vi "Automatic CE-CERT Inverter MODBUS TCP-IP Curtailment.vi"() -> ()   [LabVIEW 2018]
uses:
  09a05df4-458d-4fd2-9c33-f3dfa60df926.vi
  86d118a4-68e0-4187-aa54-a9d0a6fa2209.vi
  7d9401a8-d984-499b-98ba-350348555d74.vi
  1c5b115a-7472-46f7-9b4a-cb66c2e2ccef.vi
  14952779-31b7-4685-9780-957b5950c005.vi
  aad8307b-7fea-461e-ba7f-5a63a8c7236a.vi
  df043d8b-bec8-4485-823e-7a72ed92ff53.vi
  6303200c-3b40-4aff-b068-1284407d55db.vi
  <vilib>/Plasmionique/MB Master/MB_Master_TCP/MB_Master_TCP.lvclass
  C:/Program Files (x86)/National Instruments/LabVIEW 2018/vi.lib/Plasmionique/MB Master/MB_Master/MB_Master.lvclass
  <vilib>/Plasmionique/MB Master/MB Master.lvlib
panel:
  in  "Stop Button":bool
  in  "Send Curtailment":bool
  out "Eighth Step Time (ms)":u32
  out "Seventh Step Time (ms)":u32
  out "Sixth Step Time (ms)":u32
  out "Fifth Step Time (ms)":u32
  out "Fourth Step Time (ms)":u32
  out "Third Step Time (ms)":u32
  out "Second Step Time (ms)":u32
  out "First Step Time (ms)":u32
  out "Program Runtime (ms)":u32
  in  "Curtailment Value (28-100%)":u16
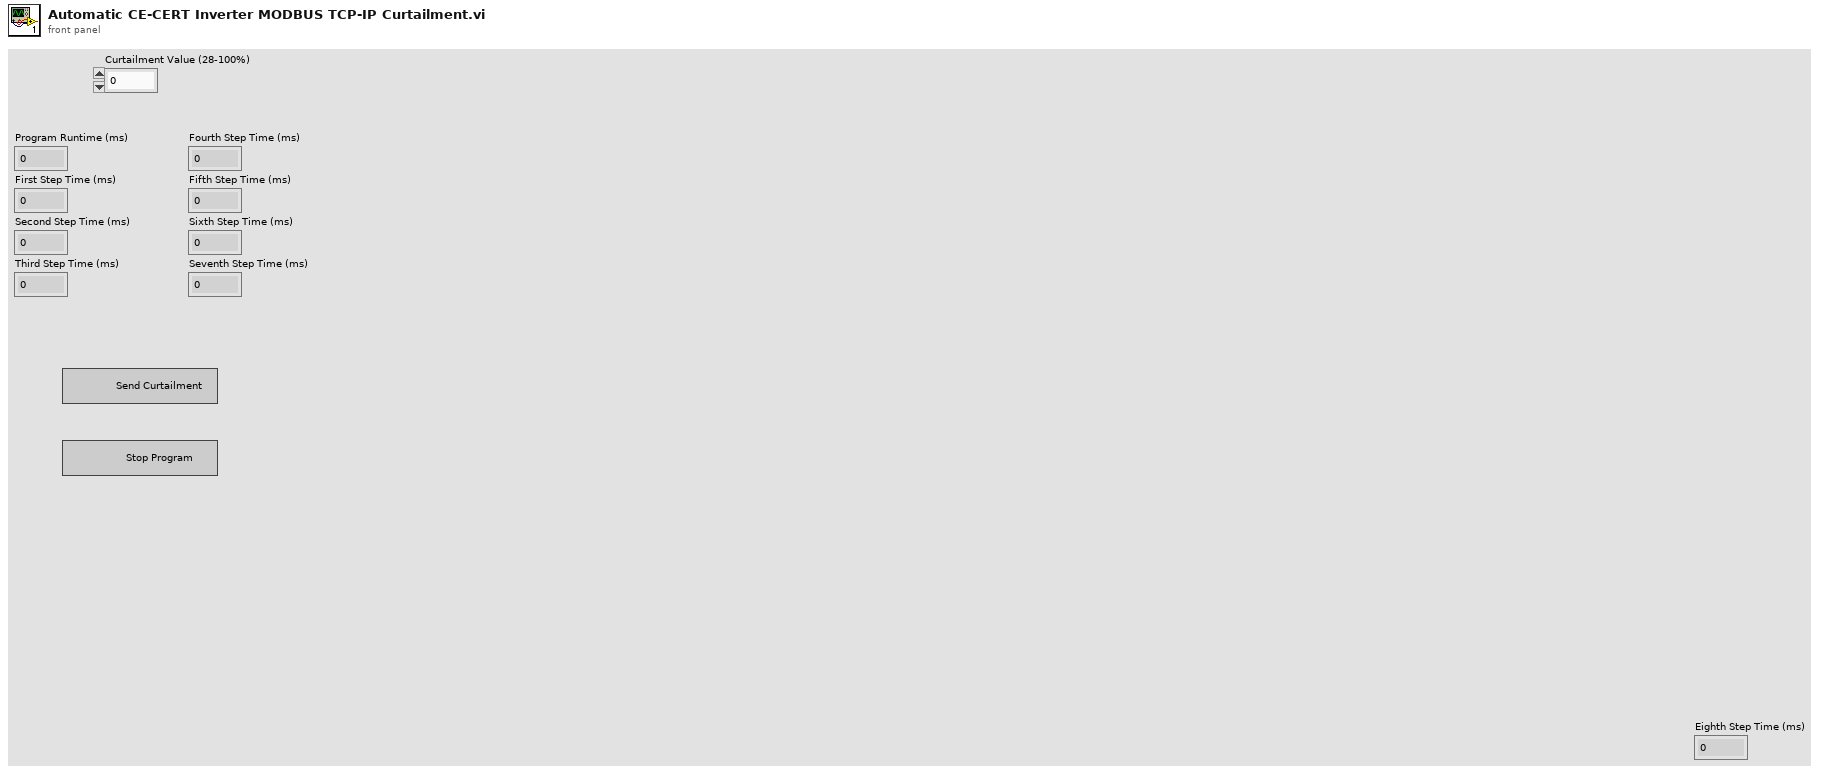
[diagram p1: front panel]
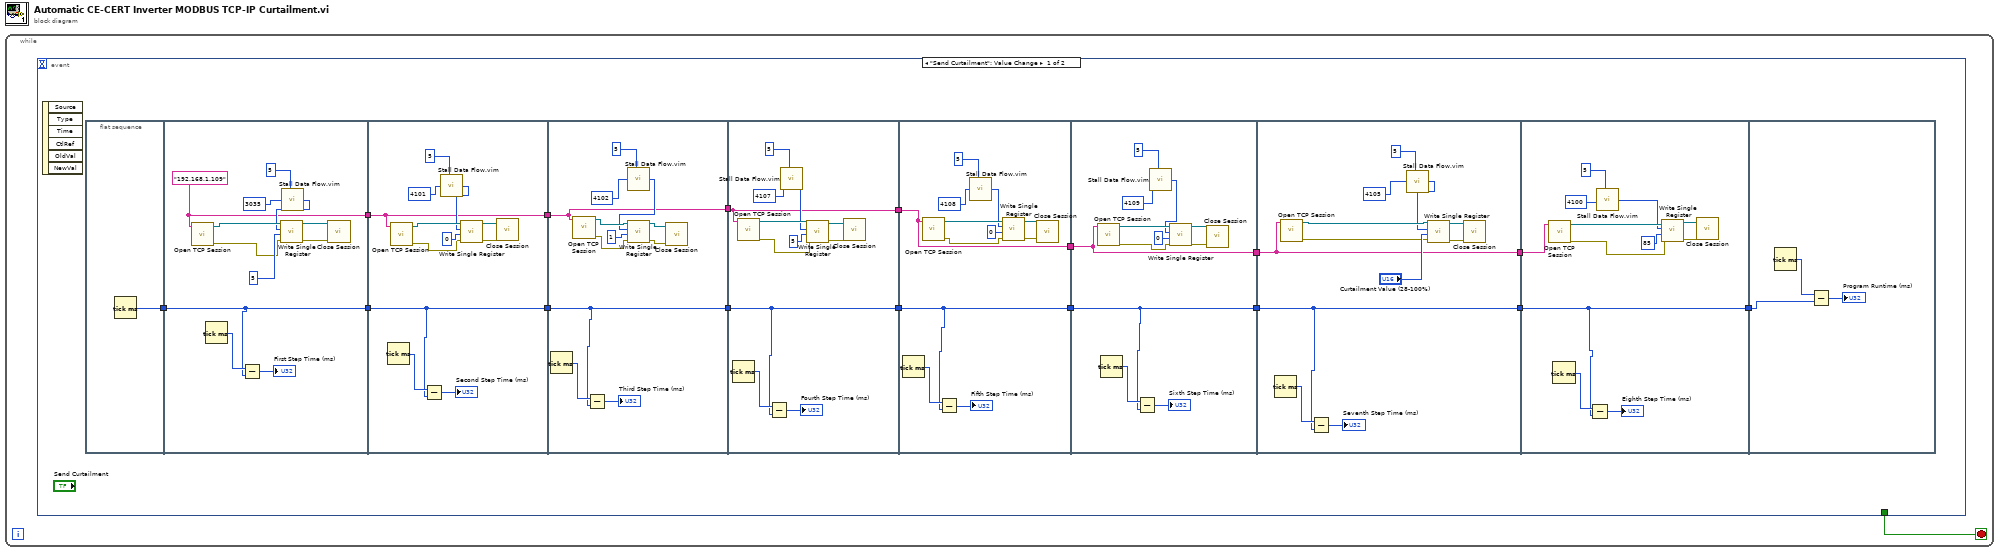
[diagram p0: block diagram]
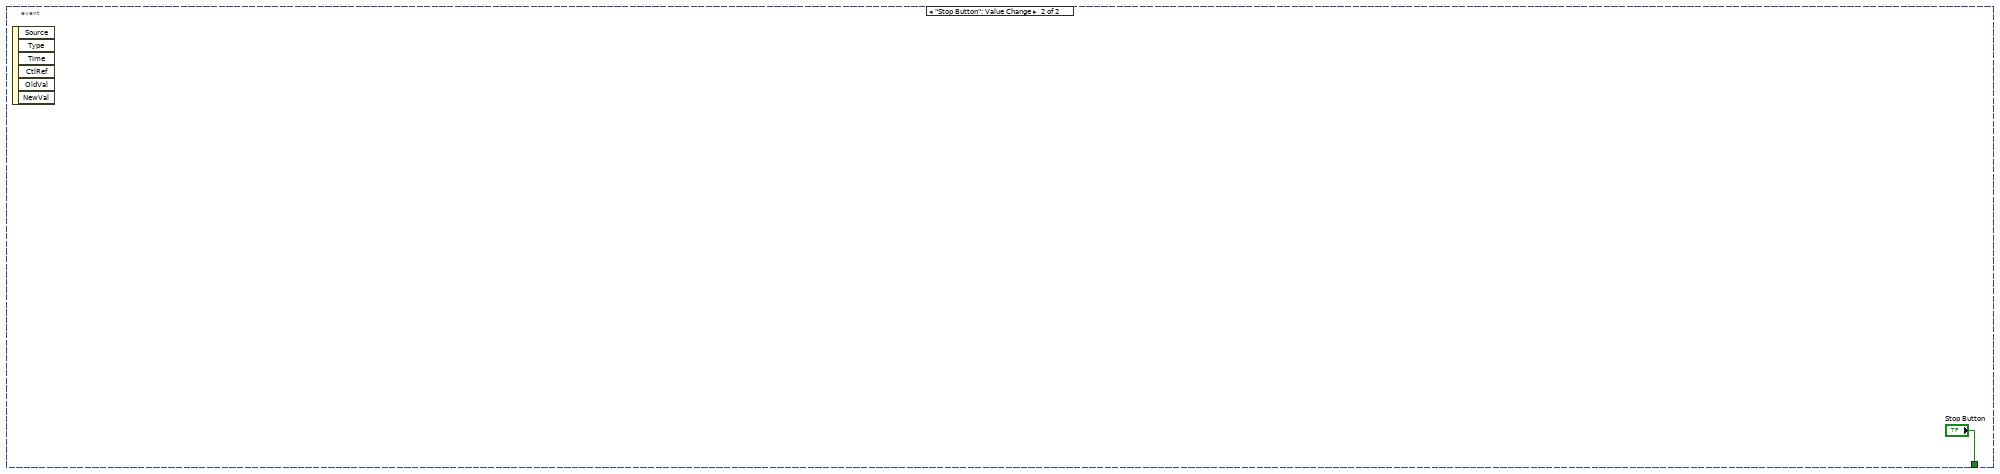
[diagram p2: hidden frame]
diagram:
  n1 = while {
    stop <- w1 stop-if-true
    n2 = event shown="[0] \"Send Curtailment\": Value Change" {
      selector: _ -> [_ _]
      dyn-events: _ -> [_ _]
      timeout: _ -> [_ _]
      tunnel: [_ "Stop Button"] -> w1
      event "Send Curtailment": Value Change {
        n3 = event-data() -> ()  [unwired: 1 in, 6 out]
        n4 = flat-sequence {
          tunnel: [w18] -> w17
          tunnel: [w21] -> w16
          tunnel: w17 -> [w21]
          tunnel: [w19] -> w15
          tunnel: [w32] -> w14
          tunnel: w16 -> [w32]
          tunnel: w15 -> [w31]
          tunnel: [w31] -> w13
          tunnel: [w44] -> w12
          tunnel: w14 -> [w44]
          tunnel: w13 -> [w43]
          tunnel: [w43] -> w11
          tunnel: [w56] -> w10
          tunnel: w12 -> [w56]
          tunnel: w11 -> [w55]
          tunnel: [w55] -> w9
          tunnel: [w68] -> w8
          tunnel: w10 -> [w68]
          tunnel: w9 -> [w67]
          tunnel: [w67] -> w7
          tunnel: [w80] -> w6
          tunnel: w8 -> [w80]
          tunnel: w7 -> [w79]
          tunnel: [w79] -> w5
          tunnel: w6 -> [w92]
          tunnel: [w92] -> w4
          tunnel: w5 -> [w91]
          tunnel: [w91] -> w3
          tunnel: w4 -> [w104]
          tunnel: [w104] -> w2
          tunnel: w3 -> [w103]
          tunnel: w2 -> [w116]
          frame #0 {
            n5 = Tick Count (ms)() -> (millisecond timer value=w18:u32)
          }
          frame #1 {
            w19 = "192.168.1.109" ("IP Address")
            n6 = call <vilib>:"Open TCP Session.vi"("IP Address"=w19) -> ("error out"=w27:errorcluster, "MB_TCP session"=w26:refnum<class "MB_Master_TCP.lvclass">)  [unwired: 9 in]
            n7 = Tick Count (ms)() -> (millisecond timer value=w22:u32)
            n8 = Subtract(x=w22, y=w21) -> (x-y=→"First Step Time (ms)":u32)
            n9 = call "Stall Data Flow.vim"("value in"=u16 3035 ("address"), "milliseconds to wait"=u32 5) -> ("value out"=w23:u16)  [unwired: 1 out]
            n10 = call <vilib>:"Write Single Register.vi"("error in (no error)"=w27, "value"=u16 5, "address"=w23, "MB session in"=w26) -> ("error out"=w28:errorcluster, "MB session out"=w29:refnum<class "MB_Master_TCP.lvclass">)  [unwired: 6 in]
            n11 = call-dynamic "Close Session.vi"("error in (no error)"=w28, "MB TCP session"=w29) -> ()  [unwired: 9 in, 1 out]
          }
          frame #2 {
            n12 = Tick Count (ms)() -> (millisecond timer value=w34:u32)
            n13 = call <vilib>:"Open TCP Session.vi"("IP Address"=w31) -> ("error out"=w40:errorcluster, "MB_TCP session"=w41:refnum<class "MB_Master_TCP.lvclass">)  [unwired: 9 in]
            n14 = Subtract(x=w34, y=w32) -> (x-y=→"Second Step Time (ms)":u32)
            n15 = call "Stall Data Flow.vim"("value in"=u16 4101 ("address"), "milliseconds to wait"=u32 5) -> ("value out"=w35:u16)  [unwired: 1 out]
            n16 = call <vilib>:"Write Single Register.vi"("error in (no error)"=w40, "value"=u16 0, "address"=w35, "MB session in"=w41) -> ("error out"=w39:errorcluster, "MB session out"=w38:refnum<class "MB_Master_TCP.lvclass">)  [unwired: 6 in]
            n17 = call-dynamic "Close Session.vi"("error in (no error)"=w39, "MB TCP session"=w38) -> ()  [unwired: 9 in, 1 out]
          }
          frame #3 {
            n18 = Tick Count (ms)() -> (millisecond timer value=w46:u32)
            n19 = call <vilib>:"Open TCP Session.vi"("IP Address"=w43) -> ("error out"=w50:errorcluster, "MB_TCP session"=w53:refnum<class "MB_Master_TCP.lvclass">)  [unwired: 9 in]
            n20 = Subtract(x=w46, y=w44) -> (x-y=→"Third Step Time (ms)":u32)
            n21 = call "Stall Data Flow.vim"("value in"=u16 4102 ("address"), "milliseconds to wait"=u32 5) -> ("value out"=w47:u16)  [unwired: 1 out]
            n22 = call <vilib>:"Write Single Register.vi"("error in (no error)"=w50, "value"=u16 1, "address"=w47, "MB session in"=w53) -> ("error out"=w52:errorcluster, "MB session out"=w51:refnum<class "MB_Master_TCP.lvclass">)  [unwired: 6 in]
            n23 = call-dynamic "Close Session.vi"("error in (no error)"=w52, "MB TCP session"=w51) -> ()  [unwired: 9 in, 1 out]
          }
          frame #4 {
            n24 = Tick Count (ms)() -> (millisecond timer value=w58:u32)
            n25 = call <vilib>:"Open TCP Session.vi"("IP Address"=w55) -> ("error out"=w62:errorcluster, "MB_TCP session"=w65:refnum<class "MB_Master_TCP.lvclass">)  [unwired: 9 in]
            n26 = Subtract(x=w58, y=w56) -> (x-y=→"Fourth Step Time (ms)":u32)
            n27 = call "Stall Data Flow.vim"("value in"=u16 4107 ("address"), "milliseconds to wait"=u32 5) -> ("value out"=w59:u16)  [unwired: 1 out]
            n28 = call <vilib>:"Write Single Register.vi"("error in (no error)"=w62, "value"=u16 5, "address"=w59, "MB session in"=w65) -> ("error out"=w64:errorcluster, "MB session out"=w63:refnum<class "MB_Master_TCP.lvclass">)  [unwired: 6 in]
            n29 = call-dynamic "Close Session.vi"("error in (no error)"=w64, "MB TCP session"=w63) -> ()  [unwired: 9 in, 1 out]
          }
          frame #5 {
            n30 = Tick Count (ms)() -> (millisecond timer value=w70:u32)
            n31 = call <vilib>:"Open TCP Session.vi"("IP Address"=w67) -> ("error out"=w74:errorcluster, "MB_TCP session"=w77:refnum<class "MB_Master_TCP.lvclass">)  [unwired: 9 in]
            n32 = Subtract(x=w70, y=w68) -> (x-y=→"Fifth Step Time (ms)":u32)
            n33 = call "Stall Data Flow.vim"("value in"=u16 4108 ("address"), "milliseconds to wait"=u32 5) -> ("value out"=w72:u16)  [unwired: 1 out]
            n34 = call <vilib>:"Write Single Register.vi"("error in (no error)"=w74, "value"=u16 0, "address"=w72, "MB session in"=w77) -> ("error out"=w76:errorcluster, "MB session out"=w75:refnum<class "MB_Master_TCP.lvclass">)  [unwired: 6 in]
            n35 = call-dynamic "Close Session.vi"("error in (no error)"=w76, "MB TCP session"=w75) -> ()  [unwired: 9 in, 1 out]
          }
          frame #6 {
            n36 = call <vilib>:"Open TCP Session.vi"("IP Address"=w79) -> ("error out"=w88:errorcluster, "MB_TCP session"=w89:refnum<class "MB_Master_TCP.lvclass">)  [unwired: 9 in]
            n37 = Tick Count (ms)() -> (millisecond timer value=w82:u32)
            n38 = Subtract(x=w82, y=w80) -> (x-y=→"Sixth Step Time (ms)":u32)
            n39 = call "Stall Data Flow.vim"("value in"=u16 4109 ("address"), "milliseconds to wait"=u32 5) -> ("value out"=w83:u16)  [unwired: 1 out]
            n40 = call <vilib>:"Write Single Register.vi"("error in (no error)"=w88, "value"=u16 0, "address"=w83, "MB session in"=w89) -> ("error out"=w86:errorcluster, "MB session out"=w87:refnum<class "MB_Master_TCP.lvclass">)  [unwired: 6 in]
            n41 = call-dynamic "Close Session.vi"("error in (no error)"=w86, "MB TCP session"=w87) -> ()  [unwired: 9 in, 1 out]
          }
          frame #7 {
            n42 = Tick Count (ms)() -> (millisecond timer value=w94:u32)
            n43 = call <vilib>:"Open TCP Session.vi"("IP Address"=w91) -> ("error out"=w98:errorcluster, "MB_TCP session"=w101:refnum<class "MB_Master_TCP.lvclass">)  [unwired: 9 in]
            n44 = Subtract(x=w94, y=w92) -> (x-y=→"Seventh Step Time (ms)":u32)
            n45 = call "Stall Data Flow.vim"("value in"=u16 4105 ("address"), "milliseconds to wait"=u32 5) -> ("value out"=w95:u16)  [unwired: 1 out]
            n46 = call <vilib>:"Write Single Register.vi"("error in (no error)"=w98, "value"="Curtailment Value (28-100%)", "address"=w95, "MB session in"=w101) -> ("error out"=w100:errorcluster, "MB session out"=w99:refnum<class "MB_Master_TCP.lvclass">)  [unwired: 6 in]
            n47 = call-dynamic "Close Session.vi"("error in (no error)"=w100, "MB TCP session"=w99) -> ()  [unwired: 9 in, 1 out]
          }
          frame #8 {
            n48 = call <vilib>:"Open TCP Session.vi"("IP Address"=w103) -> ("error out"=w110:errorcluster, "MB_TCP session"=w113:refnum<class "MB_Master_TCP.lvclass">)  [unwired: 9 in]
            n49 = Tick Count (ms)() -> (millisecond timer value=w106:u32)
            n50 = Subtract(x=w106, y=w104) -> (x-y=→"Eighth Step Time (ms)":u32)
            n51 = call "Stall Data Flow.vim"("value in"=u16 4100 ("address"), "milliseconds to wait"=u32 5) -> ("value out"=w108:u16)  [unwired: 1 out]
            n52 = call <vilib>:"Write Single Register.vi"("error in (no error)"=w110, "value"=u16 85, "address"=w108, "MB session in"=w113) -> ("error out"=w112:errorcluster, "MB session out"=w111:refnum<class "MB_Master_TCP.lvclass">)  [unwired: 6 in]
            n53 = call-dynamic "Close Session.vi"("error in (no error)"=w112, "MB TCP session"=w111) -> ()  [unwired: 9 in, 1 out]
          }
          frame #9 {
            n54 = Tick Count (ms)() -> (millisecond timer value=w117:u32)
            n55 = Subtract(x=w117, y=w116) -> (x-y=→"Program Runtime (ms)":u32)
          }
        }
      }
      event "Stop Button": Value Change {
        n56 = event-data() -> ()  [unwired: 1 in, 6 out]
      }
    }
  }
